vi "ResultsGui.vi"() -> ()   [LabVIEW 2016]
uses:
  Global/ApplicationGlobal.vi
  <vilib>/Utility/miscctls.llb/LVRowAndColumnUnsignedTypeDef.ctl
  <vilib>/Utility/miscctls.llb/LVRowAndColumnTypeDef.ctl
  tools/Config/Config.Global.vi
  Sequence/Sequence.Step.Status.ctl
  Logger/Logger.File.Properties.ctl
  Logger/Logger.File.ctl
  Sequence/Sequence.Counters.ctl
  Logger/Logger.File.Serials.ctl
  tools/Translator/Translator.Message.ctl
  <vilib>/Utility/miscctls.llb/LVBoundsTypeDef.ctl
  Sequence/Sequence.Code.SerialFormat.ctl
panel:
  out "file data in use":T1
  in  "PageIdx":i32
  out "PageSize":i32
  out "TotalSize":i32
  out "Pages":string
  in  "Btn_Next":bool
  in  "Btn_Prev":bool
  out "FileInUse":i32
  out "File content":T1[](array[typedef])
  out "_loop":i32(ring)=4
  in  "Values":i32(listbox) caption="Data"
  in  "Btn_Refresh":bool
  out "Panel":refnum<vi>
  in  "FileTree":string(tree) caption="Files"
  out "Image B":picture caption="B"
  out "Image A":picture caption="A"
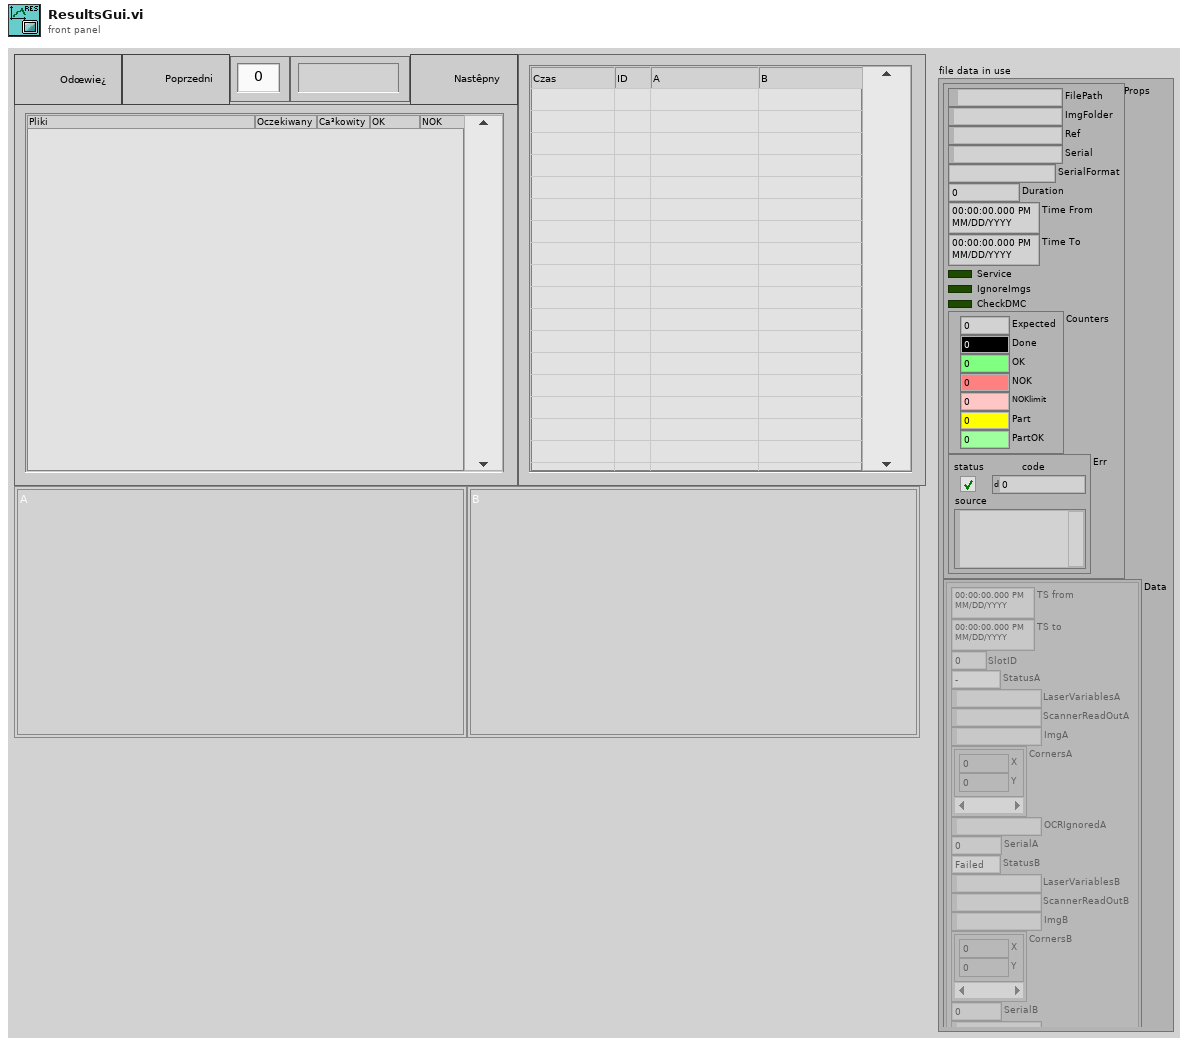
[diagram p1: front panel]
types:
  T1 = typedef "Logger.File.ctl" = cluster{"Props":T2, "Data":T5[]}
  T2 = typedef "Logger.File.Properties.ctl" = cluster{"FilePath":path, "ImgFolder":string, "Ref":string, "Serial":string, "SerialFormat":T3, "Duration":dbl, "Time From":timestamp, "Time To":timestamp, "Service":bool, "IgnoreImgs":bool, "CheckDMC":bool, "Counters":T4, "Err":errorcluster}
  T3 = typedef "Sequence.Code.SerialFormat.ctl" = enum8{"", "6 dig", "7 dig"}
  T4 = typedef "Sequence.Counters.ctl" = cluster{"Expected":u16, "Done":u16, "OK":u16, "NOK":u16, "NOKlimit":u16, "Part":u16, "PartOK":u16}
  T5 = typedef "Logger.File.Serials.ctl" = cluster{"TS from":timestamp, "TS to":timestamp, "SlotID":u8, "StatusA":T6, "LaserVariablesA":string, "ScannerReadOutA":string, "ImgA":string, "CornersA":cluster{"X":i32, "Y":i32}[], "OCRIgnoredA":string, "SerialA":u8, "StatusB":T6, "LaserVariablesB":string, "ScannerReadOutB":string, "ImgB":string, "CornersB":cluster{"X":i32, "Y":i32}[], "SerialB":u8, "OCRIgnoredB":string, "CaptionA":string, "CaptionB":string}
  T6 = typedef "Sequence.Step.Status.ctl" = enum16{"-", "Pending", "Running", "Skipped", "Passed", "Failed", "Done", "Error", "Aborted", "Stopped"}
  T7 = typedef "Translator.Message.ctl" = enum16{"-", "Event confirmed", "Log out", "Log in", "Shutdown", "Cancel", "Start", "Begin time", "End time", "Duration", "Service Mode", "Ignore Results", "Serial Format", "On", "Off", "OK", "NOK", "NOK %s", "Home", "Work", "Close", "Open", "In progress...", "Missing", "Empty", "Hardware failure", "Initial", "Default", "Total", "Out of range", "Free disk space is below 1GB - contact technician", "Error %d >> %s", "Error %d >> %s >> %s", "Msg %d >> %s", "Laser msg %d %s", "Laser cmd error %s %d", "Laser cmd failed %s", "Laser cmd warning %s", "Laser disconnected", "Laser status %s", "Laser already started", "Laser job unkonwn %s", "Laser job missing %s", "Laser job select failure %s", "Unable to start laser printing (%s)", "Unable to stop laser printing (%s)", "Laser marking aborted", "Laser marking timeout", "Unable to reset Laser Interlock (%s)", "Unable to trigger Laser. Laser not ready (%s)", "Laser job '%s' coordinates not configured", "Starting %s", "Quitting %s", "Configured", "Initializing", "Quitting", "Loading", "Loaded %d results", "Loaded %d events", "Running", "Stopped", "Summary", "Laser", "Do you want to continue?", "Do you want to delete the configuration?", "The configuration is being used by an order. Unable to delete!", "Press confirm button", "Station is not based. Do you want to exit?", "Station requires changeover. Do you want to run the test?", "Test options are not set as default. Do you want to continue?", "Formatting of WabcoNo is disabled. Do you want to continue?", "Product not detected. Do you want to continue?", "Product scan failed. Do you want to continue?", "Calibration", "Log out?", "System", "All", "IDLE", "Translating...%s", "Not found", "Alarm %s", "Run", "Skip", "Abort", "Repeat", "Please wait...", "Database disconnected", "Database disconnected - changeover disabled!", "Login to database successful", "Login to database failed: %d; %s", "Unable to check the product status of reference %d - database disconnected", "Unable to set the product status of reference %d - database disconnected", "Variant file backup %s", "Read variant (%s)", "Result", "Station armed!", "Station requires changeover!", "Select reference number...", "EMERGENCY BUTTON - press Control button", "EMERGENCY DOOR - press Control button", "Resetting Emergency...", "Unable to reset safety circuit - Emergency Button pressed", "Unable to reset safety circuit - Emergency Side Door open", "Station not based", "Station based", "Station not empty", "Station basing...", "No order", "Press Start to begin new order", "Scanning new order", "Order NOK. Correct or scan again", "Order OK. Press Accept", "Order ready", "Revolver incorrect", "Fork incorrect", "Revolver missing", "Revolver empty", "Container missing", "Offline results", "Offline statistics", "Updating statistics %.1f %%", "DMC Configurator", "Door open", "Close the front door", "Press start button", "Done. Open the front door", "Running...", "Running...%.1f %%", "Pause %s", "Pause %s. NOK container missing", "Pause %s. OK container missing", "Pause %s. Revolver empty", "Pause %s. Revolver missing", "Pause %s. Revolver incorrect", "Pause %s. Fork missing", "Pause %s. Fork incorrect", "Pause %s. Too many failures", "Pause %s. Unloading failure", "Pause %s. One slot is not working", "Pause %s. Part order is done. Empty OK container", "Pause %s. Unable to move product to slot", "Pause %s. Unable to move back product pusher", "Pause %s. Unable to lift product", "Pause %s. Unable to move back product lifter", "Pause %s. Unable to move product arm to Work", "Pause %s. Unable to move product arm to NOK", "Pause %s. Unable to move product arm to OK", "Pause %s. Unable to unsuck the NOK product", "Pause %s. Unable to drop the NOK product", "Pause %s. Product OK missing", "Pause %s. Unable to unsuck the OK product", "Pause %s. Unable to drop the OK product", "Stopping...", "File '%s' is missing", "File '%s' is broken", "File '%s' is running", "Log file started (%s)", "Log file ended (%s)", "Log file stopped (%s)", "Log file ignored (%s)", "Log file exported (%s)", "Log file export failed (%s)", "Wrong serial number in log file", "Wrong reference number in log file", "Test steps are missing", "%s = %.3f", "Process param '%s' not found in DB", "Process param '%s' wrong order", "Process param '%s' value %.3f out of limits (%.3f; %.3f)", "Step%d param '%s' not found in DB", "Step%d param '%s' wrong order", "Step%d param '%s' value %.3f out of limits (%.3f; %.3f)", "Step%d EV '%s' not found in DB", "Step%d EV '%s' wrong order", "\"%s\" not found in DB", "\"%s\" wrong order", "\"%s\" value %.3f out of limits (%.3f; %.3f)", "\"%s\" not found in software", "Process init (%s)", "Process started", "Process restarted", "Process run", "Process done", "Process done - remove OK container", "Process aborted", "Process aborted at work", "Process aborted at home", "Process error", "Process error at home", "Process error at work", "Process close", "Process pause", "Process continue", "Process door open", "Process door close", "Process pause at slot %s due to %s", "Select plate from the order to process", "Do you want to start the process?", "Do you want to continue the process?", "There is unfinished order. Do you want to put the new order?", "Product %s %d OK", "Product %s %d NOK", "Unable to unload the slot %s. Product missing in the slot", "Unable to unload the slot %s. Product already in the arm", "Unable to accept the product as OK. Product missing in slot %s", "Unable to accept the product as OK. Product could not drop into the container at slot %s", "Unable to accept the product as NOK. Product could not drop into the container at slot %s", "Scan failed. Error %s", "Scan failed. Scanner disconnected", "Scan failed. Wrong Wabco number %d, limit (%d,%d)", "Scan failed. Wrong serial number %d, limit (%d,%d)", "Scan failed. Wrong date %d, limit (%d,%d)", "Scan failed. Wrong product wabco number %d (expected %d)", "Scan failed. Wrong product serial number %d (expected > 0)", "Scan OK %s", "Scan failed. Unable to determine table position (%s)", "Scan failed. Timeout", "Tune failed. Scanner disconnected", "Tune failed. Timeout", "%s = %d", "%s = %d->%d", "Unable to set %s = %.2f - Air Pressure Inside off", "Unable to set digital output '%s' = %d", "Unable to activate air pressure inside - timeout", "Unable to activate air pressure inside - aborted", "Unable to switch on Air Main Valve - Air Pressure Inlet off", "Unable to switch on Air Main Valve - Door open", "Unable to switch off Air Main Valve - timeout", "Unable to switch off Air Main Valve - aborted", "Unable to rotate Table - timeout", "Unable to rotate Table - aborted", "Unable to rotate Table - Product Move not in Home position", "Unable to rotate Table - Air Pressure Inside off", "Unable to rotate Table - Product Lift A not in Home position", "Unable to rotate Table - Product Lift B not in Home position", "Unable to rotate Table - unlock before movement timeout", "Unable to rotate Table - lock after movement timeout", "Unable to move Table Lock to %s position - timeout", "Unable to move Table Lock to %s position - aborted", "Unable to move Table Lock to %s position - Air Pressure Inside off", "Unable to move Table Lock to %s position - Table not in position", "Unable to move Product Lift A to %s position - timeout", "Unable to move Product Lift B to %s position - timeout", "Unable to move Product Lift A to %s position - aborted", "Unable to move Product Lift B to %s position - aborted", "Unable to move Product Lift A to %s position - Air Pressure Inside off", "Unable to move Product Lift B to %s position - Air Pressure Inside off", "Unable to move Product Lift A to %s position - Table not locked", "Unable to move Product Lift B to %s position - Table not locked", "Unable to move Product Lift A to %s position - Product Arm not in Work position", "Unable to move Product Lift B to %s position - Product Arm not in Work position", "Unable to set Product Suction Gripper %s to %s - timeout", "Unable to set Product Suction Gripper %s to %s - aborted", "Unable to set Product Suction Gripper %s to %s - Air Pressure Inside off", "Unable to set Product Suction Gripper %s to %s - Table slot unkown", "Unable to move Product Arm to %s position - timeout", "Unable to move Product Arm to %s position - aborted", "Unable to move Product Arm to %s position - Air Pressure Inside off", "Unable to move Product Arm to %s position - Product Lift A not in Home position", "Unable to move Product Arm to %s position - Product Lift B not in Home position", "Unable to move Product to %s position - timeout", "Unable to move Product to %s position - aborted", "Unable to move Product to %s position - Air Pressure Inside off", "Unable to move Product to %s position - Table not in position"}
  T8 = enum8{"Enabled", "Disabled", "Disabled and Grayed Out"}
  T9 = typedef "LVRowAndColumnTypeDef.ctl" = cluster{"Row":i32, "Column":i32}
  T10 = typedef "LVRowAndColumnUnsignedTypeDef.ctl" = cluster{"Row":u32, "Column":u32}
  T11 = typedef "LVPositionTypeDef.ctl" = cluster{"Left":i32, "Top":i32}
  T12 = typedef "LVBoundsTypeDef.ctl" = cluster{"Width":u32, "Height":u32}
  T13 = enum32{"Invalid", "Standard", "Closed", "Hidden", "Minimized", "Maximized"}
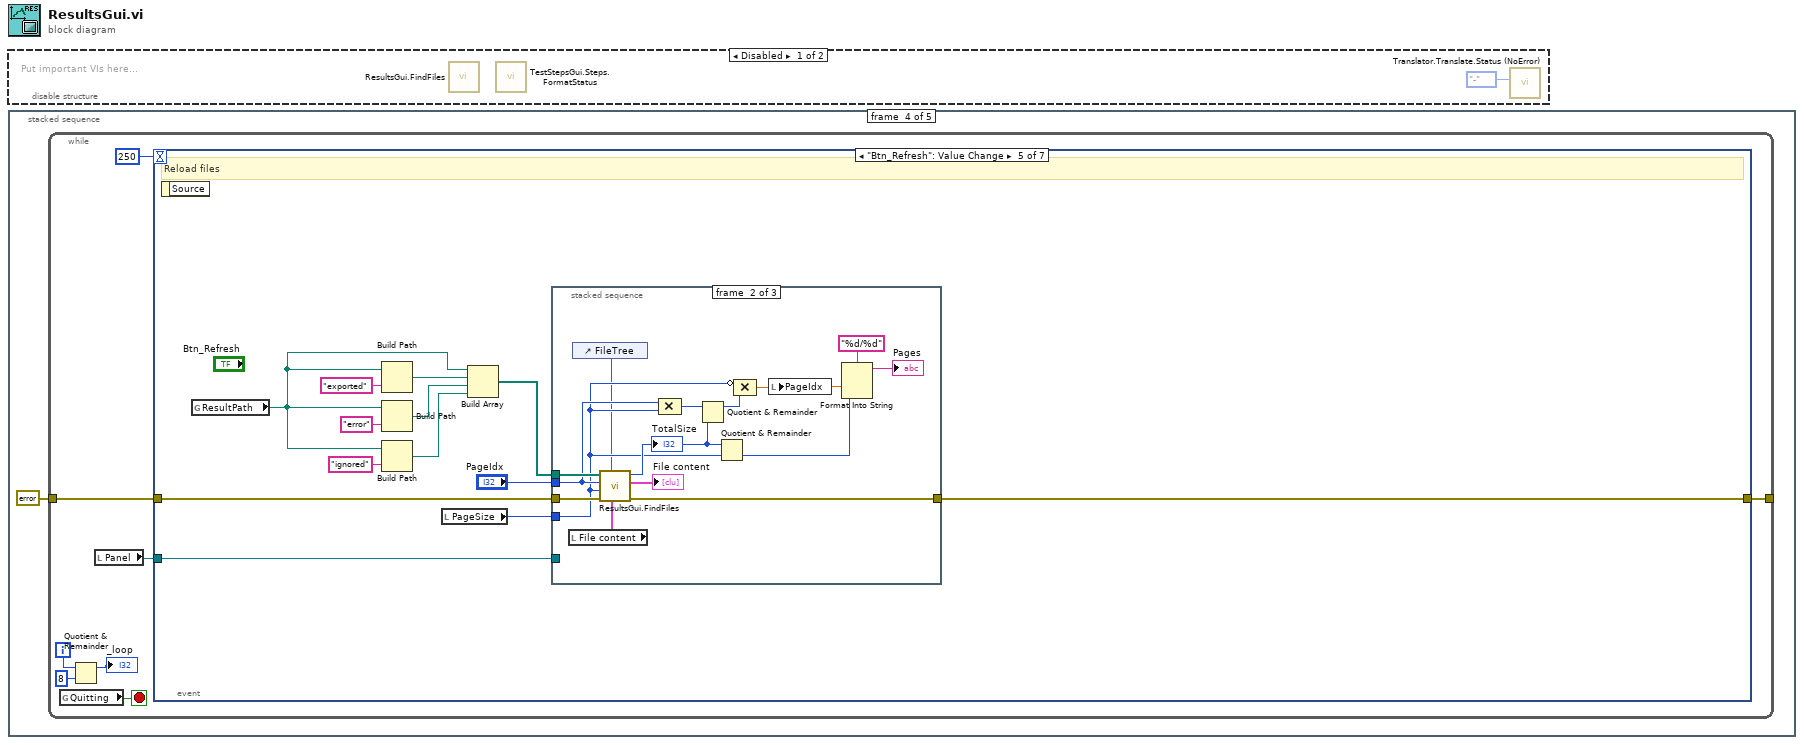
[diagram p0: block diagram]
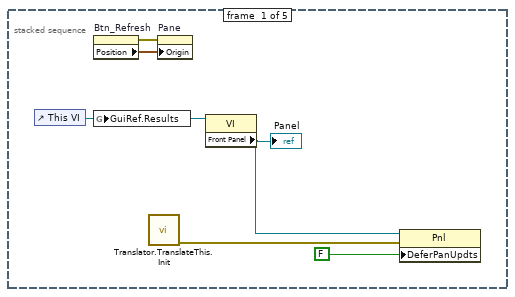
[diagram p2: hidden frame]
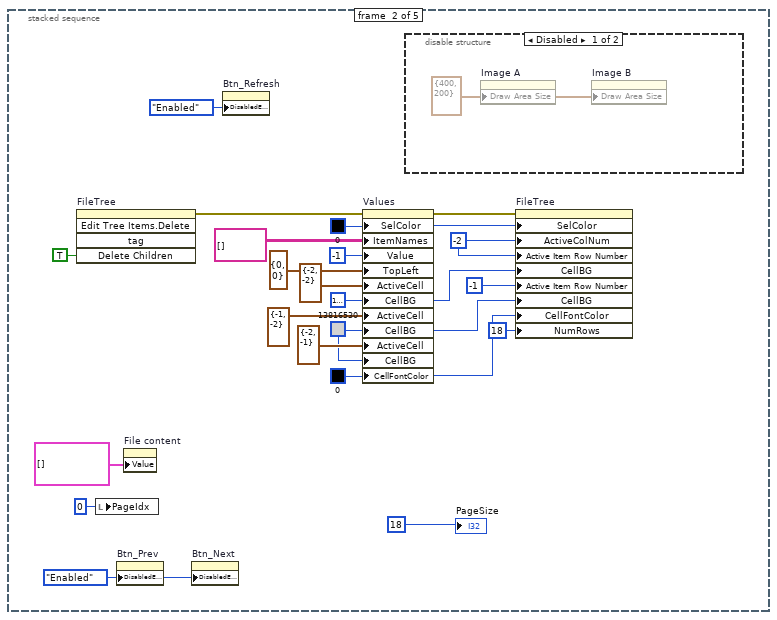
[diagram p3: hidden frame]
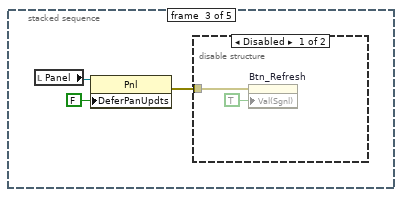
[diagram p5: hidden frame]
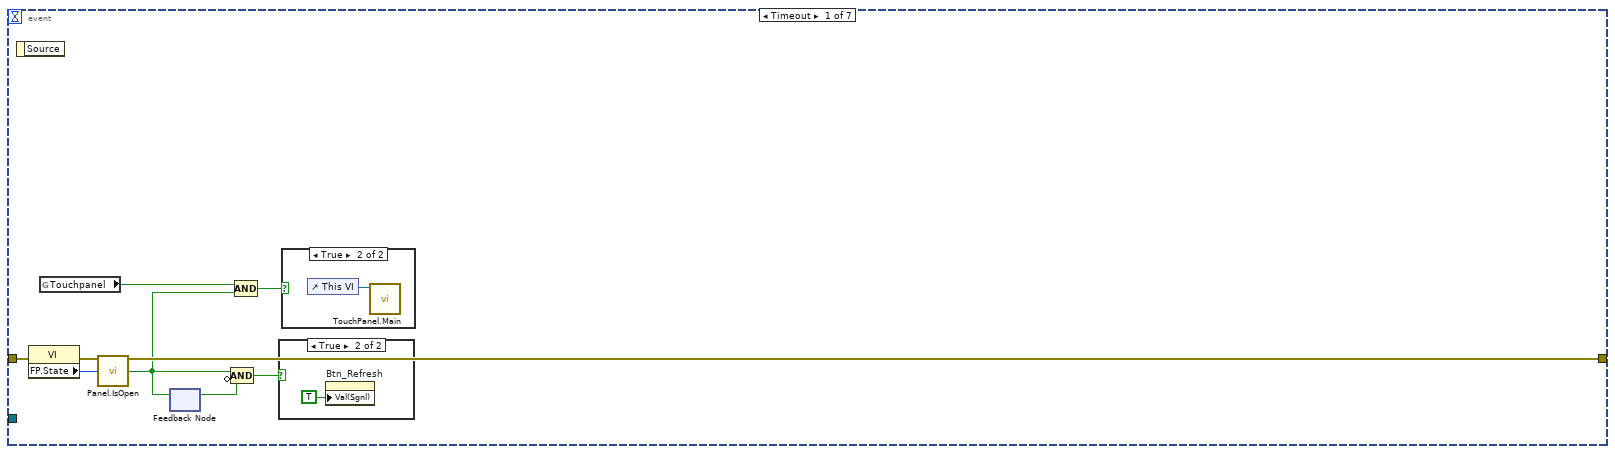
[diagram p7: hidden frame]
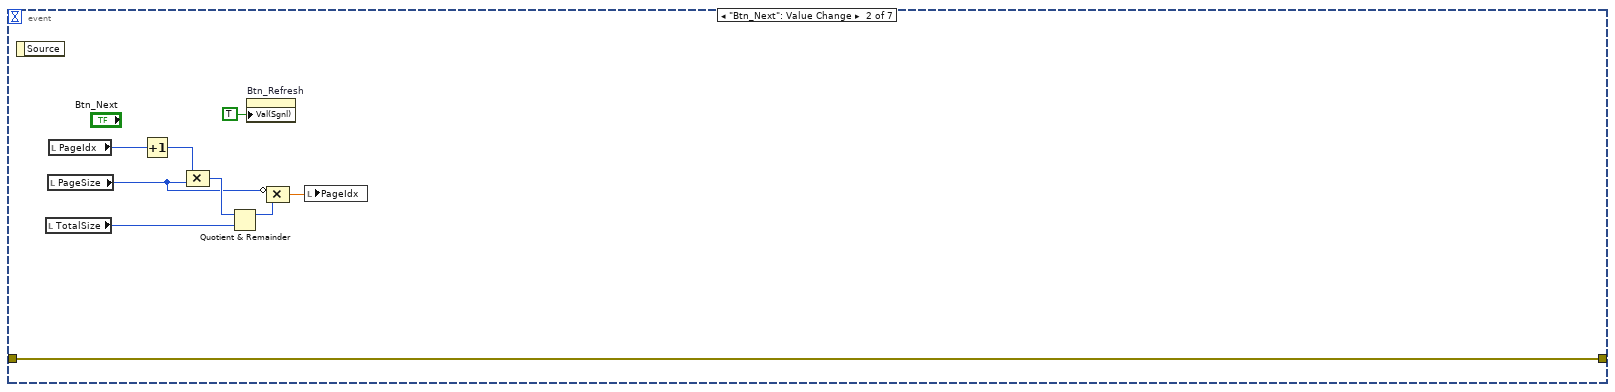
[diagram p10: hidden frame]
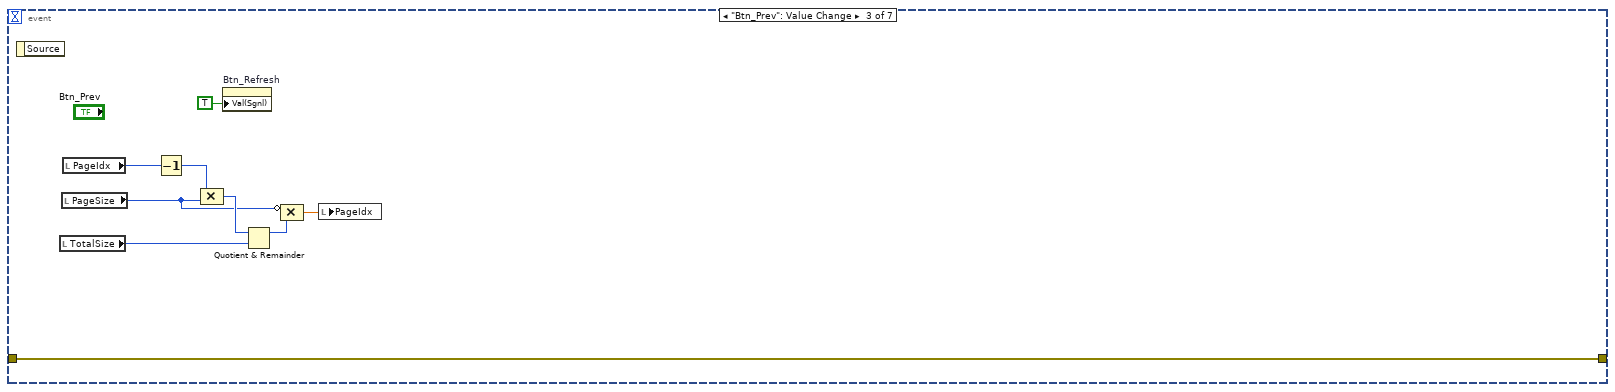
[diagram p11: hidden frame]
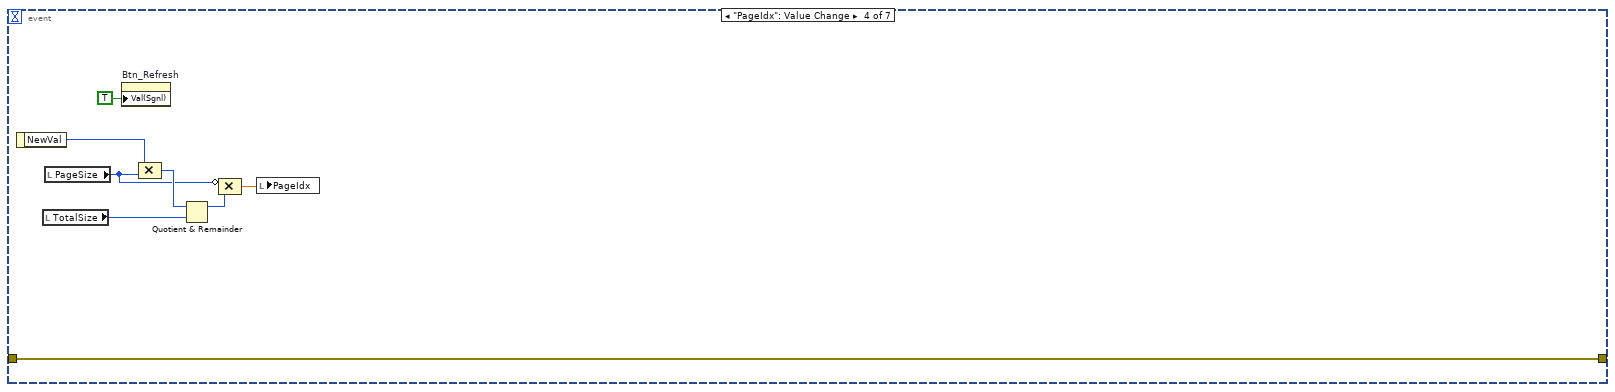
[diagram p12: hidden frame]
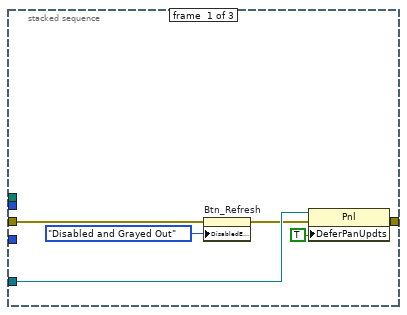
[diagram p13: hidden frame]
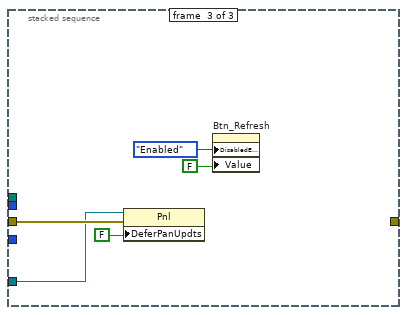
[diagram p14: hidden frame]
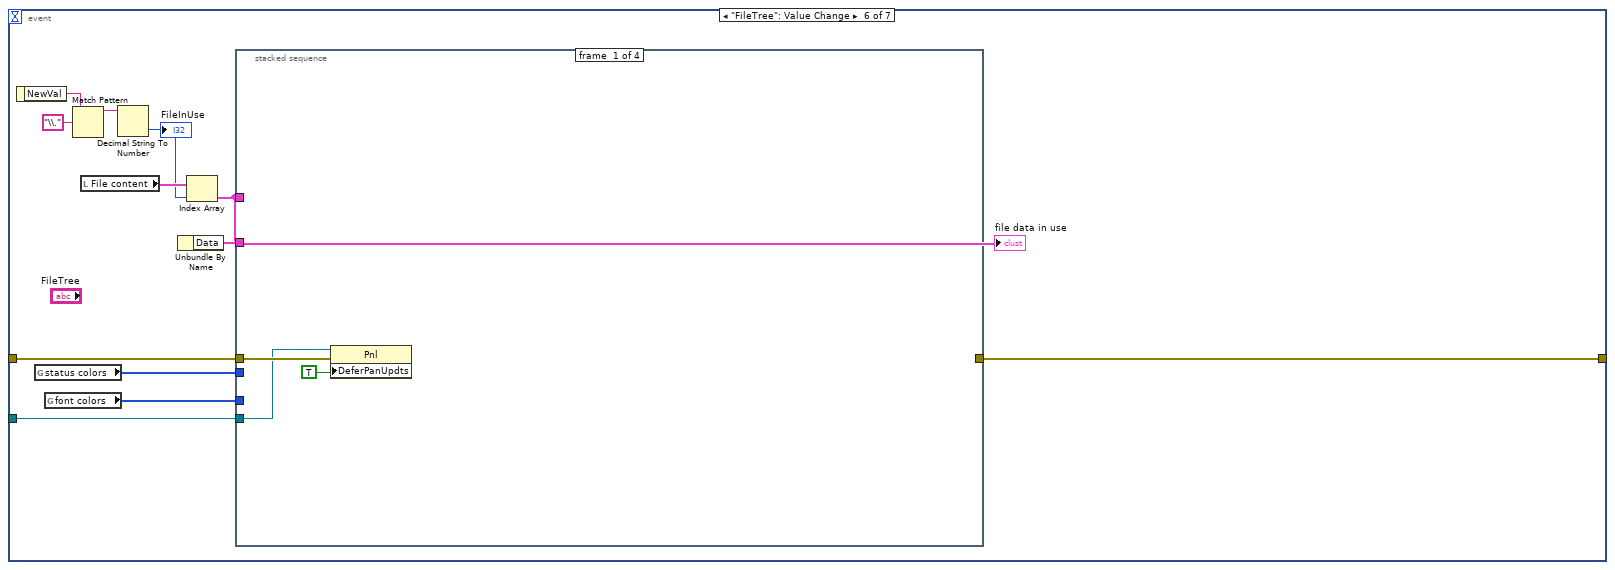
[diagram p15: hidden frame]
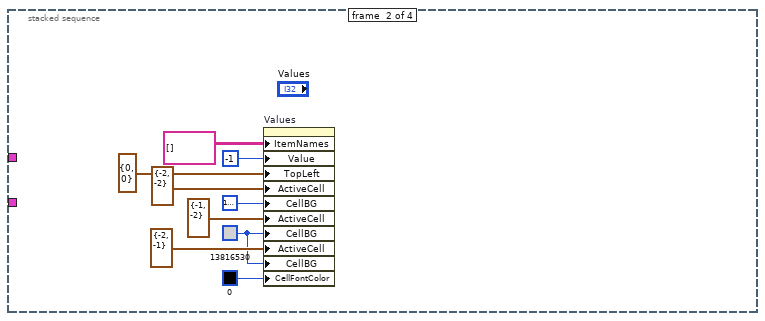
[diagram p16: hidden frame]
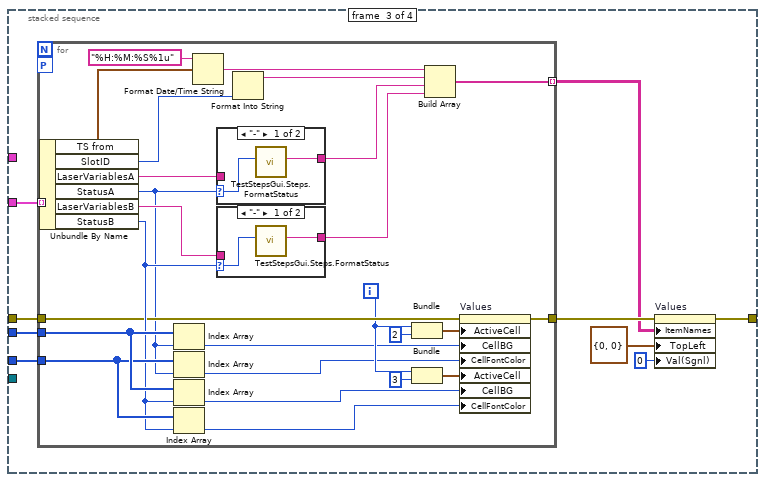
[diagram p17: hidden frame]
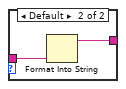
[diagram p18: hidden frame]
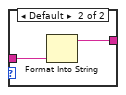
[diagram p19: hidden frame]
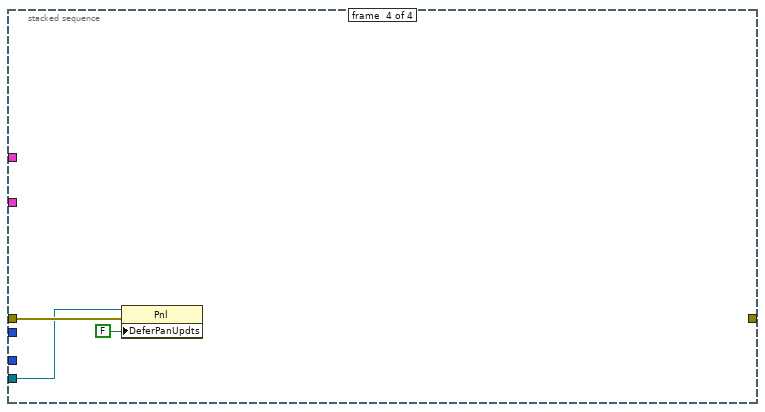
[diagram p20: hidden frame]
diagram:
  n1 = disable-structure shown="Disabled" {
    frame Disabled {
      # "Put important VIs here..."
      n2 = call "ResultsGui.FindFiles.vi"() -> ()  [unwired: 9 in, 3 out]
      n3 = call "TestStepsGui.Steps.FormatStatus.vi"() -> ()  [unwired: 11 in, 1 out]
      n4 = call "Translator.Translate.Status (NoError).vi"("msg"=Translator.Message."-") -> ()  [unwired: 10 in, 1 out]
    }
    frame Enabled {
    }
  }
  n5 = stacked-sequence {
    frame #0 {
      n6 = control-ref of="This VI"() -> (w5:refnum<vi>)
      n7 = property on="Btn_Refresh" class="Bool (strict)"() -> (error out=w7:errorcluster, "Position"=w6:T11)  [unwired: 2 in, 1 out]
      n8 = global write "ApplicationGlobal.vi" "GuiRef.Results"(w5) -> ()
      n9 = call "Translator.TranslateThis.Init.vi"() -> ("error out"=w2:errorcluster)  [unwired: 11 in]
      n10 = property on="Pane" class="Pane"(error in=w7, "Origin"=w6) -> ()  [unwired: 1 in, 2 out]
      n11 = property class="VI"(reference=w5) -> ("Front Panel"=w3:refnum<vi>)  [unwired: 1 in, 2 out]
      "Panel" <- w3
      n12 = property class="Pnl"(reference=w3, error in=w2, "DeferPanUpdts"=FALSE ("Defer Panel Updates")) -> ()  [unwired: 2 out]
    }
    frame #1 {
      w12 = u32 0
      w18 = T8."Enabled" ("Disabled")
      w14 = u32 0
      w21 = -2 ("Active Cell:Active Column Number")
      w17 = u32 13816530
      w13 = u32 16777225
      n13 = invoke on="FileTree" class="Tree (strict)" method="Edit Tree Items.Delete"("Delete Children"=TRUE ("Delete Children?")) -> (error out=w11:errorcluster)  [unwired: 4 in, 4 out]
      n14 = local write "PageIdx"(0 ("PageIdx")) -> ()
      n15 = property on="Btn_Prev" class="Bool"("DisabledEnum"=w18) -> ()  [unwired: 2 in, 2 out]
      n16 = property on="File content" class="Arr (strict)"("Value"=T1[] [] ("File content")) -> ()  [unwired: 2 in, 2 out]
      n17 = property on="Btn_Next" class="Bool"("DisabledEnum"=w18) -> ()  [unwired: 2 in, 2 out]
      n18 = property on="Btn_Refresh" class="Bool (strict)"("DisabledEnum"=T8."Enabled" ("Disabled")) -> ()  [unwired: 2 in, 2 out]
      n19 = property on="Values" class="MCListbox (strict)"(error in=w11, "SelColor"=w14, "ItemNames"=string[][] [] ("Item Names"), "Value"=-1 ("Properties"), "TopLeft"=T10 {"Row"=0, "Column"=0} ("Top Left Visible Cell"), "ActiveCell"=T9 {"Row"=-2, "Column"=-2} ("Active Cell:Active Cell"), "CellBG"=w13, "ActiveCell"=T9 {"Row"=-1, "Column"=-2} ("Active Cell:Active Cell"), "CellBG"=w17, "ActiveCell"=T9 {"Row"=-2, "Column"=-1} ("Active Cell:Active Cell"), "CellBG"=w17, "CellFontColor"=w12) -> (error out=w16:errorcluster)  [unwired: 1 in, 1 out]
      n20 = disable-structure shown="Disabled" {
        frame Disabled {
          w29 = T12 {"Width"=400, "Height"=200} ("Draw Area Size")
          n21 = property on="Image A" class="Pict"("Draw Area Size"=w29) -> ()  [unwired: 2 in, 2 out]
          n22 = property on="Image B" class="Pict"("Draw Area Size"=w29) -> ()  [unwired: 2 in, 2 out]
        }
        frame Enabled {
        }
      }
      n23 = property on="FileTree" class="Tree (strict)"(error in=w16, "SelColor"=w14, "ActiveColNum"=w21, "Active Item Row Number"=w21, "CellBG"=w13, "Active Item Row Number"=-1 ("Active Item:Row Number"), "CellBG"=w17, "CellFontColor"=w12, "NumRows"=u32 18 ("Number of Rows")) -> ()  [unwired: 1 in, 2 out]
      "PageSize" <- 18 ("PageSize")
    }
    frame #2 {
      n24 = local read "Panel"() -> (w31:refnum<vi>)
      n25 = property class="Pnl"(reference=w31, "DeferPanUpdts"=FALSE ("Defer Panel Updates")) -> (error out=w30:errorcluster)  [unwired: 1 in, 1 out]
      n26 = disable-structure shown="Disabled" {
        disable-tunnel: w30 -> [w34 _]
        frame Disabled {
          n27 = property on="Btn_Refresh" class="Bool (strict)"(error in=w34, "Val(Sgnl)"=TRUE ("Value (Signaling)")) -> ()  [unwired: 1 in, 2 out]
        }
        frame Enabled {
        }
      }
    }
    frame #3 {
      n28 = while {
        tunnel: errorcluster {"status"=FALSE, "code"=0, "source"=""} ("error out") -> [w38]
        tunnel: [w37] -> _
        i -> [w41]
        stop <- w43 stop-if-true
        n29 = global read "ApplicationGlobal.vi" "Quitting"() -> (w43:bool)
        n30 = Quotient & Remainder(x=w41, y=8) -> (x-y*floor(x/y)=→"_loop":i32)  [unwired: 1 out]
        n31 = local read "Panel"() -> (w36:refnum<vi>)
        n32 = event shown="[4] \"Btn_Refresh\": Value Change" {
          selector: _ -> [_ _ _ _ _ _ _]
          dyn-events: _ -> [_ _ _ _ _ _ _]
          timeout: 250 -> [_ _ _ _ _ _ _]
          tunnel: w38 -> [w51 w59 w70 w79 w88 w127 w222]
          tunnel: [w50 w59 w70 w79 w87 w119 w222] -> w37
          tunnel: w36 -> [_ _ _ _ w89 w122 _]
          event Timeout {
            n33 = event-data() -> ()  [unwired: 1 in, 1 out]
            n34 = property class="VI"(error in=w51) -> (error out=w50:errorcluster, "FP.State"=w46:T13)  [unwired: 1 in, 1 out]
            n35 = global read "Config.Global.vi" "Touchpanel"() -> (w49:bool)
            n36 = call "Panel.IsOpen.vi"("FP State"=w46) -> ("Open?"=w44:bool)
            n37 = feedback-in #1(w44) -> ()
            n38 = feedback #1() -> (w48:bool)  [unwired: 1 in]
            n39 = Compound Arithmetic op=AND(w44, invert w48) -> (w47:bool)
            n40 = Compound Arithmetic op=AND(w49, w44) -> (w45:bool)
            n41 = case shown="True" w47 {
              frame False {
              }
              frame True {
                n42 = property on="Btn_Refresh" class="Bool (strict)"("Val(Sgnl)"=TRUE ("Value (Signaling)")) -> ()  [unwired: 2 in, 2 out]
              }
            }
            n43 = case shown="True" w45 {
              frame False {
              }
              frame True {
                n44 = control-ref of="This VI"() -> (w53:refnum<vi>)
                n45 = call "TouchPanel.Main.vi"("VI ref"=w53) -> ()  [unwired: 8 in, 3 out]
              }
            }
          }
          event "Btn_Next": Value Change {
            n46 = event-data() -> ()  [unwired: 1 in, 1 out]
            n47 = local read "TotalSize"() -> (w57:i32)
            n48 = local read "PageSize"() -> (w55:i32)
            n49 = local read "PageIdx"() -> (w62:i32)
            n50 = Increment(x=w62) -> (x+1=w61:i32)
            n51 = Compound Arithmetic op=MULTIPLY(w61, w55) -> (w58:i32)
            n52 = Quotient & Remainder(x=w58, y=w57) -> (x-y*floor(x/y)=w56:i32)  [unwired: 1 out]
            n53 = property on="Btn_Refresh" class="Bool (strict)"("Val(Sgnl)"=TRUE ("Value (Signaling)")) -> ()  [unwired: 2 in, 2 out]
            n54 = Compound Arithmetic op=MULTIPLY(invert w55, w56) -> (w54:dbl)
            n55 = local write "PageIdx"(w54) -> ()
          }
          event "Btn_Prev": Value Change {
            n56 = event-data() -> ()  [unwired: 1 in, 1 out]
            n57 = local read "TotalSize"() -> (w66:i32)
            n58 = local read "PageSize"() -> (w64:i32)
            n59 = local read "PageIdx"() -> (w69:i32)
            n60 = Decrement(x=w69) -> (x-1=w68:i32)
            n61 = Compound Arithmetic op=MULTIPLY(w68, w64) -> (w67:i32)
            n62 = property on="Btn_Refresh" class="Bool (strict)"("Val(Sgnl)"=TRUE ("Value (Signaling)")) -> ()  [unwired: 2 in, 2 out]
            n63 = Quotient & Remainder(x=w67, y=w66) -> (x-y*floor(x/y)=w65:i32)  [unwired: 1 out]
            n64 = Compound Arithmetic op=MULTIPLY(invert w64, w65) -> (w63:dbl)
            n65 = local write "PageIdx"(w63) -> ()
          }
          event "PageIdx": Value Change {
            n66 = event-data() -> ("NewVal"=w72:i32)  [unwired: 1 in]
            n67 = local read "TotalSize"() -> (w77:i32)
            n68 = local read "PageSize"() -> (w75:i32)
            n69 = property on="Btn_Refresh" class="Bool (strict)"("Val(Sgnl)"=TRUE ("Value (Signaling)")) -> ()  [unwired: 2 in, 2 out]
            n70 = Compound Arithmetic op=MULTIPLY(w72, w75) -> (w78:i32)
            n71 = Quotient & Remainder(x=w78, y=w77) -> (x-y*floor(x/y)=w76:i32)  [unwired: 1 out]
            n72 = Compound Arithmetic op=MULTIPLY(invert w75, w76) -> (w74:dbl)
            n73 = local write "PageIdx"(w74) -> ()
          }
          event "Btn_Refresh": Value Change {
            # "Reload files"
            n74 = event-data() -> ()  [unwired: 1 in, 1 out]
            n75 = global read "ApplicationGlobal.vi" "ResultPath"() -> (w81:path)
            n76 = Build Path(base path=w81, name or relative path="exported") -> (appended path=w86:path)
            n77 = Build Path(base path=w81, name or relative path="error") -> (appended path=w84:path)
            n78 = Build Path(base path=w81, name or relative path="ignored") -> (appended path=w85:path)
            n79 = local read "PageSize"() -> (w83:i32)
            n80 = Build Array(w81, w86, w84, w85) -> (w80:path[])
            n81 = stacked-sequence {
              tunnel: w80 -> [_ w112 _]
              tunnel: w88 -> [w95 w111 w116]
              tunnel: [_ w110 _] -> w87
              tunnel: w89 -> [w96 _ w115]
              tunnel: "PageIdx" -> [_ w108 _]
              tunnel: w83 -> [_ w103 _]
              frame #0 {
                n82 = property on="Btn_Refresh" class="Bool (strict)"(error in=w95, "DisabledEnum"=T8."Disabled and Grayed Out" ("Disabled")) -> (error out=w94:errorcluster)  [unwired: 1 in, 1 out]
                n83 = property class="Pnl"(reference=w96, error in=w94, "DeferPanUpdts"=TRUE ("Defer Panel Updates (F)")) -> ()  [unwired: 2 out]
              }
              frame #1 {
                n84 = local read "File content"() -> (w99:T1[])
                n85 = control-ref of="FileTree"() -> (w100:refnum<vi>)
                n86 = call "ResultsGui.FindFiles.vi"("File content prev"=w99, "File list tree"=w100, "error in (no error)"=w111, "PageSize (100)"=w103, "PageIdx"=w108, "Paths"=w112) -> ("error out"=w110:errorcluster, "File content"=→"File content":T1[], "TotalSize"=w106:i32)  [unwired: 3 in]
                "TotalSize" <- w106
                n87 = Compound Arithmetic op=MULTIPLY(w108, w103) -> (w107:i32)
                n88 = Quotient & Remainder(x=w107, y=w106) -> (x-y*floor(x/y)=w102:i32)  [unwired: 1 out]
                n89 = Quotient & Remainder(x=w106, y=w103) -> (floor(x/y)=w98:i32)  [unwired: 1 out]
                n90 = Compound Arithmetic op=MULTIPLY(invert w103, w102) -> (w101:dbl)
                n91 = local write "PageIdx"(w101) -> ()
                n92 = Format Into String(format string="%d/%d", w101, w98) -> (resulting string=→"Pages":string)  [unwired: 2 in, 1 out]
              }
              frame #2 {
                n93 = property class="Pnl"(reference=w115, error in=w116, "DeferPanUpdts"=FALSE ("Defer Panel Updates (F)")) -> ()  [unwired: 2 out]
                n94 = property on="Btn_Refresh" class="Bool (strict)"("DisabledEnum"=T8."Enabled" ("Disabled"), "Value"=FALSE ("Btn_Refresh")) -> ()  [unwired: 2 in, 2 out]
              }
            }
          }
          event "FileTree": Value Change {
            n95 = event-data() -> ("NewVal"=w121:string)  [unwired: 1 in]
            n96 = global read "ApplicationGlobal.vi" "status colors"() -> (w123:u32[])
            n97 = global read "ApplicationGlobal.vi" "font colors"() -> (w120:u32[])
            n98 = Match Pattern(string=w121, regular expression="\\.") -> (before substring=w124:string)  [unwired: 1 in, 3 out]
            n99 = local read "File content"() -> (w128:T1[])
            n100 = Decimal String To Number(string=w124) -> (number=w125:i32)  [unwired: 2 in, 1 out]
            "FileInUse" <- w125
            n101 = Index Array(array=w128, index=w125) -> (element=w118:T1)
            "file data in use" <- w118
            n102 = Unbundle By Name(w118) -> ("Data"=w126:T5[])
            n103 = stacked-sequence {
              tunnel: [_ _ w143 _] -> w119
              tunnel: w127 -> [w131 _ w148 w186]
              tunnel: w126 -> [_ _ w147 _]
              tunnel: w122 -> [w130 _ _ w185]
              tunnel: w123 -> [_ _ w150 _]
              tunnel: w118 -> [_ _ _ _]
              tunnel: w120 -> [_ _ w149 _]
              frame #0 {
                n104 = property class="Pnl"(reference=w130, error in=w131, "DeferPanUpdts"=TRUE ("Defer Panel Updates (F)")) -> ()  [unwired: 2 out]
              }
              frame #1 {
                w133 = u32 13816530
                n105 = property on="Values" class="MCListbox (strict)"("ItemNames"=string[][] [] ("Item Names"), "Value"=-1 ("Properties"), "TopLeft"=T10 {"Row"=0, "Column"=0} ("Top Left Visible Cell"), "ActiveCell"=T9 {"Row"=-2, "Column"=-2} ("Active Cell:Active Cell"), "CellBG"=u32 16777225, "ActiveCell"=T9 {"Row"=-1, "Column"=-2} ("Active Cell:Active Cell"), "CellBG"=w133, "ActiveCell"=T9 {"Row"=-2, "Column"=-1} ("Active Cell:Active Cell"), "CellBG"=w133, "CellFontColor"=u32 0) -> ()  [unwired: 2 in, 2 out]
              }
              frame #2 {
                n106 = for {
                  tunnel: w147 -> [w154] mode=indexing
                  tunnel: w150 -> [w174]
                  tunnel: w149 -> [w173]
                  tunnel: [w171] -> w142 mode=indexing
                  tunnel: w148 -> [w165]
                  tunnel: [w164] -> w146
                  workers-P: _ -> [_]
                  i -> [w163]
                  n107 = Unbundle By Name(w154) -> ("TS from"=w156:timestamp, "SlotID"=w153:u8, "LaserVariablesA"=w175:string, "StatusA"=w151:T6, "LaserVariablesB"=w152:string, "StatusB"=w170:T6)
                  n108 = Index Array(array=w174, index=w151) -> (element=w162:u32)
                  n109 = Index Array(array=w173, index=w151) -> (element=w161:u32)
                  n110 = Index Array(array=w174, index=w170) -> (element=w160:u32)
                  n111 = Index Array(array=w173, index=w170) -> (element=w159:u32)
                  n112 = Format Date/Time String(time format string (%c)="%H:%M:%S%1u", seconds (now)=w156) -> (date/time string=w155:string)  [unwired: 1 in]
                  n113 = case shown="\"-\"" w151 {
                    selector: w151 -> [w182 _]
                    tunnel: w175 -> [_ w184]
                    tunnel: [w181 w183] -> w172
                    frame "-" {
                      n114 = call "TestStepsGui.Steps.FormatStatus.vi"("Status"=w182) -> ("Status str"=w181:string)  [unwired: 10 in]
                    }
                    frame Default {
                      n115 = Format Into String(w184) -> (resulting string=w183:string)  [unwired: 3 in, 1 out]
                    }
                  }
                  n116 = case shown="\"-\"" w170 {
                    selector: w170 -> [w178 _]
                    tunnel: w152 -> [_ w180]
                    tunnel: [w177 w179] -> w158
                    frame "-" {
                      n117 = call "TestStepsGui.Steps.FormatStatus.vi"("Status"=w178) -> ("Status str"=w177:string)  [unwired: 10 in]
                    }
                    frame Default {
                      n118 = Format Into String(w180) -> (resulting string=w179:string)  [unwired: 3 in, 1 out]
                    }
                  }
                  n119 = Format Into String(w153) -> (resulting string=w176:string)  [unwired: 3 in, 1 out]
                  n120 = Bundle(w163, 2) -> (w166:cluster{i32, i32})  [unwired: 1 in]
                  n121 = Bundle(w163, 3) -> (w168:cluster{i32, i32})  [unwired: 1 in]
                  n122 = Build Array(w155, w176, w172, w158) -> (w171:string[])
                  n123 = property on="Values" class="MCListbox (strict)"(error in=w165, "ActiveCell"=w166, "CellBG"=w162, "CellFontColor"=w161, "ActiveCell"=w168, "CellBG"=w160, "CellFontColor"=w159) -> (error out=w164:errorcluster)  [unwired: 1 in, 1 out]
                }
                n124 = property on="Values" class="MCListbox (strict)"(error in=w146, "ItemNames"=w142, "TopLeft"=T10 {"Row"=0, "Column"=0} ("Top Left Visible Cell"), "Val(Sgnl)"=0 ("Value (Signaling)")) -> (error out=w143:errorcluster)  [unwired: 1 in, 1 out]
              }
              frame #3 {
                n125 = property class="Pnl"(reference=w185, error in=w186, "DeferPanUpdts"=FALSE ("Defer Panel Updates")) -> ()  [unwired: 2 out]
              }
            }
          }
          event "Values": Value Change {
            n126 = event-data() -> ("NewVal"=w219:i32)  [unwired: 1 in]
            n127 = local read "file data in use"() -> (w212:T1)
            n128 = Unbundle By Name(w212) -> ("Data"=w223:T5[])  [unwired: 2 out]
            n129 = global read "ApplicationGlobal.vi" "LogPath"() -> (w209:path)
            n130 = Index Array(array=w223, index=w219) -> (element=w216:T5)
            n131 = Unbundle By Name(w216) -> ("ImgA"=w211:string, "CornersA"=w218:cluster{"X":i32, "Y":i32}[], "ImgB"=w210:string, "CornersB"=w217:cluster{"X":i32, "Y":i32}[], "LaserVariablesA"=w208:string, "ScannerReadOutA"=w200:string, "OCRIgnoredA"=w196:string, "LaserVariablesB"=w205:string, "ScannerReadOutB"=w198:string, "OCRIgnoredB"=w190:string)  [unwired: 1 out]
            n132 = Build Path(base path=w209, name or relative path="scanner") -> (appended path=w220:path)
            n133 = Decimal String To Number(string=w196) -> (number=w195:i32)  [unwired: 2 in, 1 out]
            n134 = Decimal String To Number(string=w190) -> (number=w191:i32)  [unwired: 2 in, 1 out]
            n135 = Equal To 0?(x=w195) -> (x = 0?=w194:bool)
            n136 = Equal To 0?(x=w191) -> (x = 0?=w192:bool)
            n137 = Not(x=w194) -> (.not. x?=w193:bool)
            n138 = Not(x=w192) -> (.not. x?=w189:bool)
            n139 = call "StringToArray.vi"("spreadsheet string"=w200) -> ("array"=w199:string[])
            n140 = call "StringToArray.vi"("spreadsheet string"=w208) -> ("array"=w207:string[])
            n141 = call "StringToArray.vi"("spreadsheet string"=w205) -> ("array"=w206:string[])
            n142 = call "StringToArray.vi"("spreadsheet string"=w198) -> ("array"=w197:string[])
            n143 = call "CreateCaptionText.vi"("Side"="A", "IgnoreOCR"=w193, "ScannerReadOut"=w199, "LaserVariables"=w207) -> ("Caption"=w202:string)  [unwired: 6 in, 1 out]
            n144 = call "CreateCaptionText.vi"("Side"="B", "IgnoreOCR"=w189, "ScannerReadOut"=w197, "LaserVariables"=w206) -> ("Caption"=w201:string)  [unwired: 6 in, 1 out]
            n145 = Build Path(base path=w220, name or relative path=w211) -> (appended path=w221:path)
            n146 = Build Path(base path=w220, name or relative path=w210) -> (appended path=w215:path)
            n147 = call "Sequence.Prod.LoadImg.vi"("corners"=w217, "path"=w215) -> ("img"=→"Image B":picture)  [unwired: 9 in]
            n148 = call "Sequence.Prod.LoadImg.vi"("corners"=w218, "path"=w221) -> ("img"=→"Image A":picture)  [unwired: 9 in]
            n149 = property on="Image A" class="Pict"("Caption.Text"=w202) -> ()  [unwired: 2 in, 2 out]
            n150 = property on="Image B" class="Pict"("Caption.Text"=w201) -> ()  [unwired: 2 in, 2 out]
          }
        }
      }
    }
    frame #4 {
      n151 = global read "ApplicationGlobal.vi" "ResultPath"() -> (w224:path)
      n152 = Build Path(base path=w224, name or relative path="exported") -> (appended path=w226:path)
      n153 = call "Translator.TranslateThis.Exit.vi"() -> ("error out"=w228:errorcluster)  [unwired: 11 in]
      n154 = Build Array(w224, w226) -> (w225:path[])
      n155 = local read "Panel"() -> (w229:refnum<vi>)
      n156 = for {
        tunnel: w225 -> [w231] mode=indexing
        tunnel: [w230] -> _
        workers-P: _ -> [_]
        n157 = List Folder(path=w231, pattern="*.tdms_index" ("string")) -> (path out=w233:path, filenames=w234:string[], error out=w232:errorcluster)  [unwired: 2 in, 1 out]
        n158 = for {
          tunnel: w233 -> [w240]
          tunnel: w234 -> [w239] mode=indexing
          tunnel: [w237] -> w230
          tunnel: w232 -> [w236]
          workers-P: _ -> [_]
          n159 = Build Path(base path=w240, name or relative path=w239) -> (appended path=w238:path)
          n160 = Delete(path (use dialog)=w238, error in=w236) -> (error out=w237:errorcluster)  [unwired: 3 in, 2 out]
        }
      }
      n161 = Close Reference(reference=w229, error in (no error)=w228) -> ()  [unwired: 1 out]
    }
  }
